vi "dummy encoder speed calculation (non FPGA).vi"(6 "encoder fixed offest":sgl, 9 "angle pulse":u32, 11 "speed pulse":u32) -> (1 "calculated angle (radians)":sgl, 3 "calculated speed (rad/tick)":sgl)   [LabVIEW 2018]
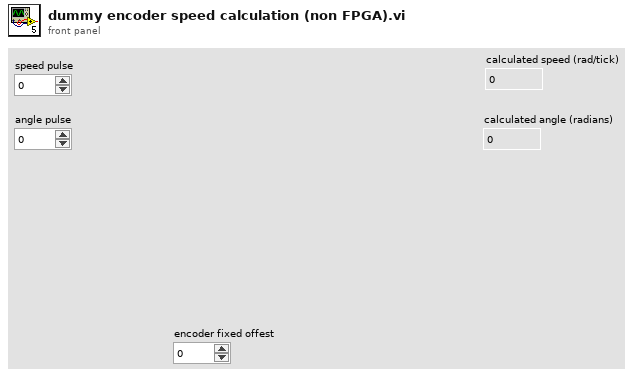
[diagram p1: front panel]
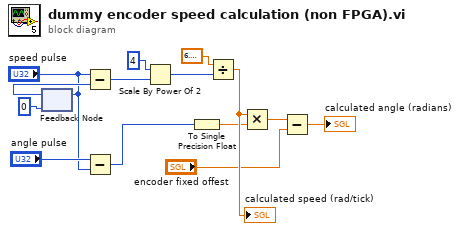
[diagram p0: block diagram]
diagram:
  n1 = feedback-in #1("speed pulse") -> ()
  n2 = feedback #1(u32 0 ("speed pulse")) -> (w6:u32)
  n3 = Subtract(x="speed pulse", y=w6) -> (x-y=w4:u32)
  n4 = Subtract(x="angle pulse", y="speed pulse") -> (x-y=w8:u32)
  n5 = Scale By Power Of 2(n=i16 4, x=w4) -> (x*2^n=w2:u32)
  n6 = To Single Precision Float(number=w8) -> (single precision float=w1:sgl)
  n7 = Divide(x=sgl 6.2831855, y=w2) -> (x/y=w13:sgl)
  "calculated speed (rad/tick)" <- w13
  n8 = Multiply(x=w13, y=w1) -> (x*y=w12:sgl)
  n9 = Subtract(x=w12, y="encoder fixed offest") -> (x-y=→"calculated angle (radians)":sgl)
